vi "JSONRPC-ArrayToString_String.vi"(11 "Array":string[](array[string])) -> (3 "Output":string)   [LabVIEW 2020]
panel:
  # "ArrayToString_String"
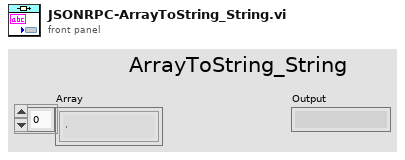
[diagram p1: front panel]
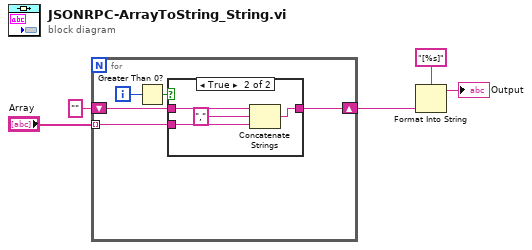
[diagram p0: block diagram]
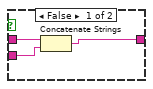
[diagram p2: hidden frame]
diagram:
  n1 = for {
    tunnel: "Array" -> [w6] mode=indexing
    shift-right: [w10] -> w4
    shift-left: "" -> [w9]
    i -> [w8]
    n2 = Greater Than 0?(x=w8) -> (x > 0?=w7:bool)
    n3 = case shown="True" w7 {
      tunnel: w6 -> [w11 w15]
      tunnel: [w13 w14] -> w10
      tunnel: w9 -> [w12 w17]
      frame False {
        n4 = Concatenate Strings(w12, w11) -> (w13:string)
      }
      frame True {
        n5 = Concatenate Strings(w17, "," ("string"), w15) -> (w14:string)
      }
    }
  }
  n6 = Format Into String(format string="[%s]", w4) -> (resulting string=→"Output":string)  [unwired: 2 in, 1 out]
